vi "Retrieve Housekeeping.vi"(8 "error in":errorcluster, 10 "LF AI":refnum<k21>, 11 "CRDS Data In":refnum<class "cCRDS Data.lvclass">) -> (0 "error out":errorcluster, 2 "Data Out":sgl[][](array[numeric]), 3 "CRDS Data Out":refnum<class "cCRDS Data.lvclass">)   [LabVIEW 2015, in "cCRDS.lvclass"]
uses:
  cCRDS.lvclass
  Data/cCRDS Data.lvclass
  Controls/Flags.ctl
  <vilib>/DAQmx/read.llb/DAQmx Read (Analog 2D DBL NChan NSamp).vi
  <vilib>/DAQmx/miscellaneous.llb/DAQmx Fill In Error Info.vi
  Reusable/General/Temperature/Convert R to T - DBL Array.vi
  Data/Write Pressure.vi
  Data/Write vData.vi
  Data/Write Humidifier T.vi
  Data/Write Thermistor T.vi
  Reusable/CRDS/Data/Main/Write filter.vi
  Reusable/Data/Write measTime.vi
  Reusable/General/Temperature/Temperature.lvlib
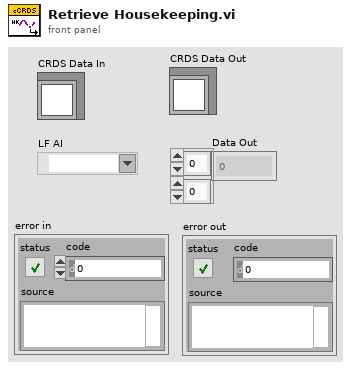
[diagram p1: front panel]
types:
  T1 = typedef "Flags.ctl" = enum8{"Autospeaker", "Link cycles", "Autofilter", "O3 Cal", "Filter Position"}
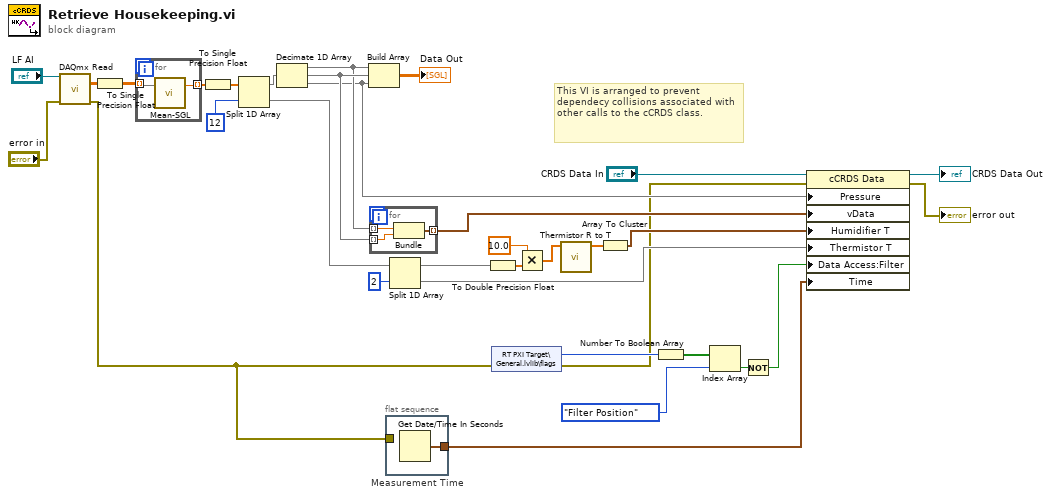
[diagram p0: block diagram]
diagram:
  # "This VI is arranged to prevent dependecy collisions associated with other calls to the cCRDS class."
  n1 = call-poly <vilib>:"DAQmx Read.vi"("task/channels in"="LF AI", "error in"="error in") -> ("data"=w9:dbl[][], "error out"=w4:errorcluster)  [unwired: 11 in, 1 out]
  n2 = To Single Precision Float(number=w9) -> (single precision float=w10:sgl[][])
  n3 = for {
    tunnel: w10 -> [w35] mode=indexing
    tunnel: [w34] -> w24 mode=indexing
    n4 = call "Mean-SGL.vi"("Data"=w35) -> ("Mean"=w34:sgl)  [unwired: 2 in]
  }
  n5 = To Single Precision Float(number=w24) -> (single precision float=w25:sgl[])
  n6 = Split 1D Array(array=w25, index=12) -> (first subarray=w20:sgl[], second subarray=w22:sgl[])
  n7 = Decimate 1D Array(w20) -> (w32:sgl[], w33:sgl[], w16:sgl[])
  n8 = Build Array(w32, w33, w16) -> (→"Data Out":sgl[][])
  n9 = for {
    tunnel: w32 -> [w38] mode=indexing
    tunnel: w33 -> [w37] mode=indexing
    tunnel: [w36] -> w19 mode=indexing
    n10 = Bundle("Mean"=w38, "Mean"=w37) -> (w36:cluster{"Mean":sgl, "Mean":sgl})  [unwired: 1 in]
  }
  n11 = flat-sequence "Measurement Time" {
    tunnel: [w39] -> w3
    tunnel: w4 -> [_]
    frame #0 {
      n12 = Get Date/Time In Seconds() -> (seconds since 1Jan1904=w39:timestamp)
    }
  }
  n13 = Split 1D Array(array=w22, index=2) -> (first subarray=w30:sgl[], second subarray=w17:sgl[])
  n14 = To Double Precision Float(number=w30) -> (double precision float=w31:dbl[])
  n15 = shared-variable "RT PXI Target\\General.lvlib\\flags"(error in=w4) -> (w15:u8, error out=w8:errorcluster)
  n16 = Multiply(x=10.0, y=w31) -> (x*y=w29:dbl[])
  n17 = call-poly "Thermistor R to T.vi"("R"=w29) -> ("T"=w27:dbl[])  [unwired: 9 in, 1 out]
  n18 = Array To Cluster(array=w27) -> (cluster=w18:cluster{"T[0]":dbl, "T[1]":dbl})
  n19 = Number To Boolean Array(number=w15) -> (Boolean array=w14:bool[])
  n20 = Index Array(array=w14, index=Flags."Filter Position" ("Flags")) -> (element=w6:bool)
  n21 = Not(x=w6) -> (.not. x?=w5:bool)
  n22 = property class="cCRDS Data"(reference="CRDS Data In", error in=w8, "Pressure"=w16, "vData"=w19, "Humidifier T"=w18, "Thermistor T"=w17, "Data Access:Filter"=w5, "Time"=w3) -> (reference out=→"CRDS Data Out":refnum<class "cCRDS Data.lvclass">, error out=→"error out":errorcluster)
